vi "Handle Value Change.vi"(5 "VolatusAPI":refnum<class "VolatusAPI.lvclass">, 7 "CtlRef":refnum<vi>, 8 "error in (no error)":errorcluster, 9 "NewVal":variant, 10 "OldVal":variant, 11 "ImageButtonControl in":refnum<class "ImageButtonControl.lvclass">) -> (0 "error out":errorcluster, 3 "ImageButtonControl out":refnum<class "ImageButtonControl.lvclass">)   [LabVIEW 2023, in "VolatusGUIElements.lvlib" / "ImageButtonControl.lvclass"]
uses:
  ImageButtonControl.lvclass
  Volatus/VolatusAPI/VolatusAPI.lvclass
  messages/CmdDigital/Data.ctl
  ImageButtonControl.lvclass/ImageButtonControl.ctl
  messages/CmdDigital/Class/Msg.lvclass/Msg.ctl
  Volatus/VolatusAPI/VolatusAPI.lvclass/VolatusAPI.ctl
  messages/CmdDigital/Class/Msg.lvclass
  lv-vecto/Vecto/TCPMessageService/Send Message.vi
  <vilib>/Utility/error.llb/Error Cluster From Error Code.vi
  lv-protoc/LV-Proto/Message/Message.lvclass
  messages/CmdDigital/CmdDigital.lvlib
  VolatusGUI/GUI Element/GUI Element.lvclass
  messages/CmdDigitalMultiple/Class/Msg.lvclass
  C:/dev/volatus/mts-volatus-super/libs/lv-volatus/messages/CmdDigitalMultiple/Class/Msg.lvclass
  C:/dev/volatus/mts-volatus-super/libs/lv-protoc/LV-Proto/Message/Message.lvclass
  C:/dev/volatus/mts-volatus-super/libs/lv-volatus/VolatusGUI/GUI Element/GUI Element.lvclass
  C:/dev/volatus/mts-volatus-super/libs/lv-volatus/VolatusGUIElements/ImageButtonControl/ImageButtonControl.lvclass
  C:/dev/volatus/mts-volatus-super/libs/lv-volatus/VolatusGUI/OnValueChangeHandler/OnValueChangeHandler.lvclass
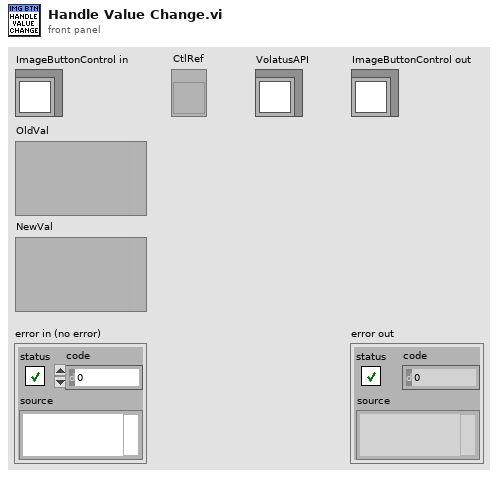
[diagram p1: front panel]
types:
  T1 = typedef "CmdDigital.lvlib/Data.ctl" = cluster{"channel":string, "value":bool}
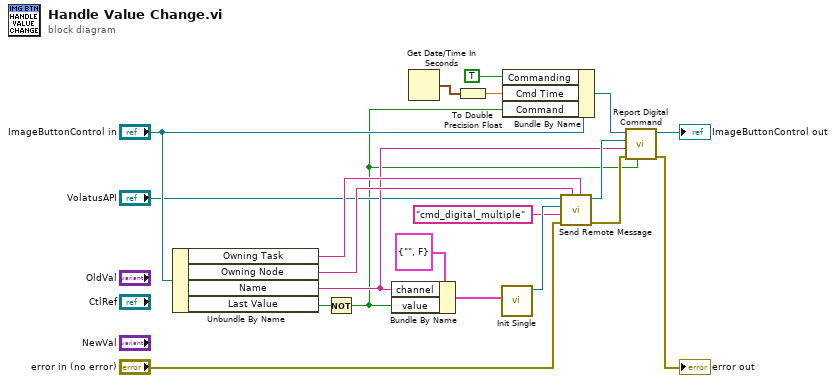
[diagram p0: block diagram]
diagram:
  n1 = Unbundle By Name("ImageButtonControl in") -> ("Owning Task"=w12:string, "Owning Node"=w11:string, "Name"=w8:string, "Last Value"=w2:bool)
  n2 = Not(x=w2) -> (.not. x?=w1:bool)
  n3 = Bundle By Name(cluster=T1 {"channel"="", "value"=FALSE} ("Data"), "channel"=w8, "value"=w1) -> (w19:T1)
  n4 = Get Date/Time In Seconds() -> (seconds since 1Jan1904=w15:timestamp)
  n5 = To Double Precision Float(number=w15) -> (double precision float=w14:dbl)
  n6 = call "Init Single.vi"("value"=w19) -> ("Msg out"=w18:refnum<class "Msg.lvclass">)  [unwired: 10 in]
  n7 = Bundle By Name(cluster="ImageButtonControl in", "Commanding"=TRUE, "Cmd Time"=w14, "Command"=w1) -> (w16:refnum<class "ImageButtonControl.lvclass">)
  n8 = call "Send Remote Message.vi"("Target Task (None)"=w12, "Target Name"=w11, "error in (no error)"="error in (no error)", "Message Type"="cmd_digital_multiple", "Message"=w18, "VolatusAPI in"="VolatusAPI") -> ("error out"=w10:errorcluster, "VolatusAPI out"=w9:refnum<class "VolatusAPI.lvclass">)  [unwired: 4 in]
  n9 = call "Report Digital Command.vi"("Value"=w1, "error in (no error)"=w10, "Name"=w8, "VolatusAPI in"=w9, "GUI Element in"=w16) -> ("error out"=→"error out":errorcluster, "GUI Element out"=→"ImageButtonControl out":refnum<class "ImageButtonControl.lvclass">)  [unwired: 5 in]
